vi "datearray_folder_creation.vi"(8 "error in":errorcluster, 11 "Cluster":T1={"path_Orig"=path "", "bo_Empty_Orig"=TRUE, "bo_exist_Orig"=TRUE, "path_Destin"=path "", "bo_Empty_Dest"=TRUE, "bo_exist_Dest"=TRUE, "bool_Erase"=FALSE, "arr_cl_lastmod_path"=[]}) -> (0 "error out":errorcluster, 3 "arr_copiedfiles":path[](array[path]))   [LabVIEW 2026]
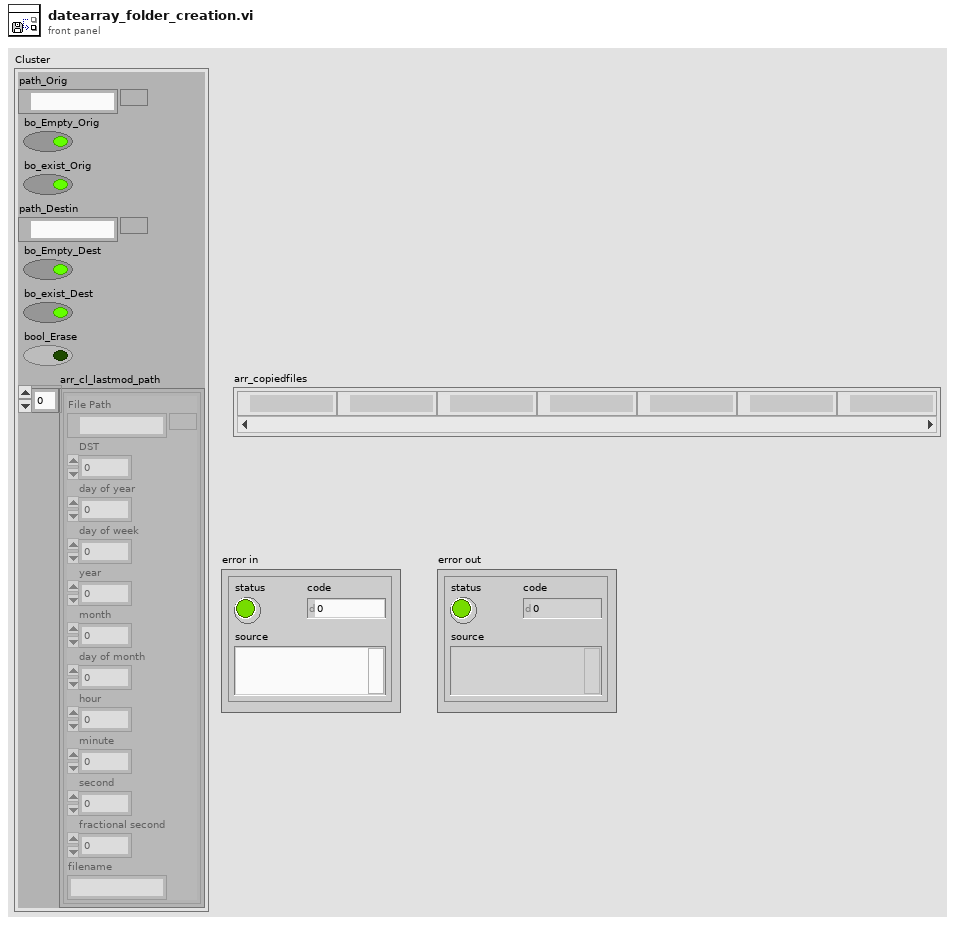
[diagram p1: front panel]
types:
  T1 = cluster{"path_Orig":path, "bo_Empty_Orig":bool, "bo_exist_Orig":bool, "path_Destin":path, "bo_Empty_Dest":bool, "bo_exist_Dest":bool, "bool_Erase":bool, "arr_cl_lastmod_path":cluster{"File Path":path, "DST":i32, "day of year":i32, "day of week":i32, "year":i32, "month":i32, "day of month":i32, "hour":i32, "minute":i32, "second":i32, "fractional second":dbl, "filename":string}[]}
  T2 = cluster{"File Path":path, "DST":i32, "day of year":i32, "day of week":i32, "year":i32, "month":i32, "day of month":i32, "hour":i32, "minute":i32, "second":i32, "fractional second":dbl, "filename":string}[]
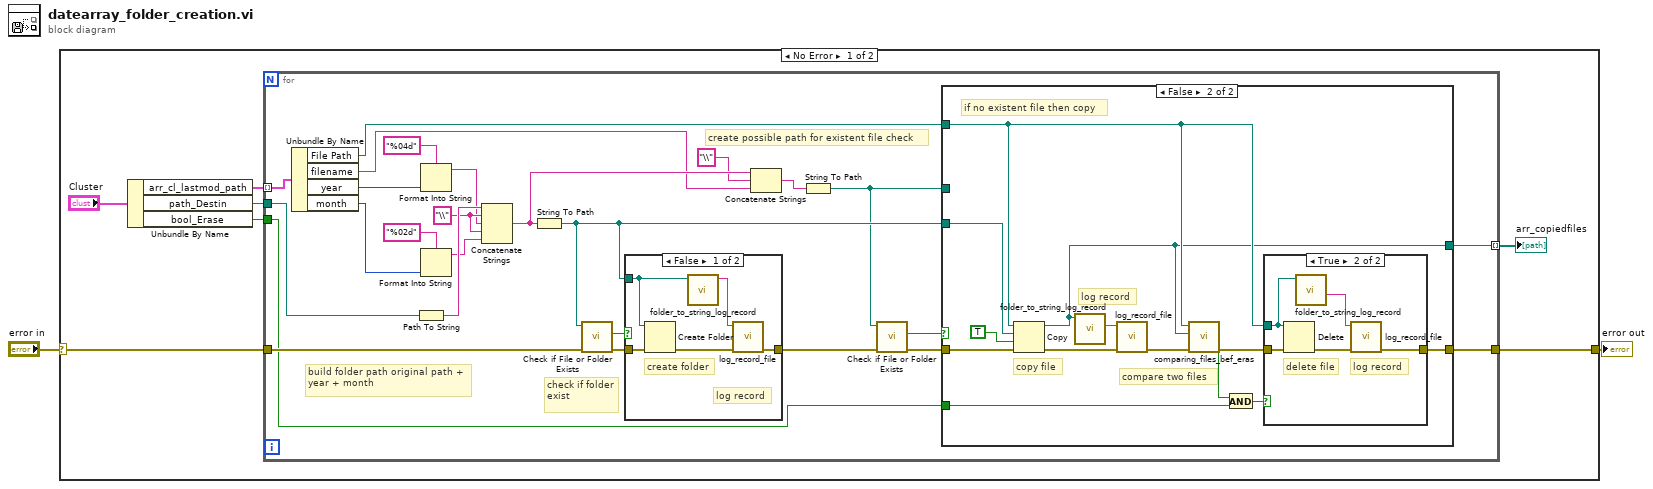
[diagram p0: block diagram]
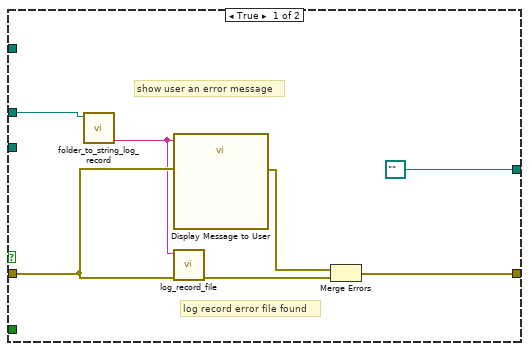
[diagram p2: hidden frame]
diagram:
  n1 = case shown="No Error" "error in" {
    selector: "error in" -> [w9 w68]
    tunnel: [w7 w68] -> w1
    frame No Error {
      n2 = Unbundle By Name("Cluster") -> ("arr_cl_lastmod_path"=w5:T2, "path_Destin"=w8:path, "bool_Erase"=w3:bool)
      n3 = for {
        tunnel: w8 -> [w34]
        tunnel: w9 -> [w32]
        tunnel: [w22] -> w7
        tunnel: [w20] -> w6 mode=indexing
        tunnel: w5 -> [w21] mode=indexing
        tunnel: w3 -> [w16]
        w33 = "\\"
        # "create possible path for existent file check"
        # "check if folder exist"
        # "build folder path original path + year + month"
        n4 = Unbundle By Name(w21) -> ("File Path"=w15:path, "filename"=w11:string, "year"=w26:i32, "month"=w29:i32)
        n5 = Path To String(path=w34) -> (string=w35:string)
        n6 = Format Into String(format string="%04d", w26) -> (resulting string=w25:string)  [unwired: 2 in, 1 out]
        n7 = Format Into String(format string="%02d", w29) -> (resulting string=w24:string)  [unwired: 2 in, 1 out]
        n8 = Concatenate Strings(w35, w33, w25, w33, w24) -> (w13:string)
        n9 = String To Path(string=w13) -> (path=w23:path)
        n10 = call <vilib>:"Check if File or Folder Exists.vi"("error in (no error)"=w32, "path"=w23) -> ("error out"=w30:errorcluster, "file or folder exists?"=w31:bool)  [unwired: 7 in, 1 out]
        n11 = case shown="False" w31 {
          tunnel: w30 -> [w66 w67]
          tunnel: [w64 w67] -> w19
          tunnel: w23 -> [w62 _]
          frame False {
            # "log record"
            # "create folder"
            n12 = Create Folder(path (use dialog)=w62, error in=w66) -> (error out=w65:errorcluster)  [unwired: 1 in, 2 out]
            n13 = call "folder_to_string_log_record.vi"("File Path"=w62) -> ("str_foldercreat"=w63:string)  [unwired: 7 in, 3 out]
            n14 = call "log_record_file.vi"("error in"=w65, "st_LogEvent"=w63) -> ("error out"=w64:errorcluster)  [unwired: 9 in]
          }
          frame True {
          }
        }
        n15 = Concatenate Strings(w13, "\\", w11) -> (w14:string)
        n16 = String To Path(string=w14) -> (path=w10:path)
        n17 = call <vilib>:"Check if File or Folder Exists.vi"("error in (no error)"=w19, "path"=w10) -> ("error out"=w18:errorcluster, "file or folder exists?"=w17:bool)  [unwired: 7 in, 1 out]
        n18 = case shown="False" w17 {
          tunnel: w18 -> [w40 w55]
          tunnel: w23 -> [_ w53]
          tunnel: [w41 w52] -> w22
          tunnel: w15 -> [_ w47]
          tunnel: [path "" ("new path") w46] -> w20
          tunnel: w16 -> [_ w49]
          tunnel: w10 -> [w38 _]
          frame True {
            # "show user an error message"
            # "log record error file found"
            n19 = call "folder_to_string_log_record.vi"("File Path"=w38) -> ("str_fileerrror"=w37:string)  [unwired: 7 in, 3 out]
            n20 = call "Display Message to User"("error in (no error)"=w40, "Message"=w37) -> ("error out"=w39:errorcluster)  [unwired: 8 in, 1 out]
            n21 = call "log_record_file.vi"("error in"=w40, "st_LogEvent"=w37) -> ("error out"=w42:errorcluster)  [unwired: 9 in]
            n22 = Merge Errors(w39, w42) -> (w41:errorcluster)
          }
          frame False {
            # "compare two files"
            # "if no existent file then copy"
            # "log record"
            # "copy file"
            n23 = Copy(8:w55, 9:TRUE, 10:w53, 11:w47) -> (0:w51:errorcluster, 3:w46:path)  [unwired: 1 in, 1 out]
            n24 = call "folder_to_string_log_record.vi"("File Path"=w46) -> ("str_filecopyed"=w50:string)  [unwired: 7 in, 3 out]
            n25 = call "log_record_file.vi"("error in"=w51, "st_LogEvent"=w50) -> ("error out"=w44:errorcluster)  [unwired: 9 in]
            n26 = call "comparing_files_bef_eras.vi"("error in"=w44, "path_filecopied"=w46, "path_fileorigin"=w47) -> ("error out"=w43:errorcluster, "bol_equals"=w45:bool)  [unwired: 7 in]
            n27 = And(x=w45, y=w49) -> (x .and. y?=w48:bool)
            n28 = case shown="True" w48 {
              tunnel: [w56 w59] -> w52
              tunnel: w43 -> [w56 w61]
              tunnel: w47 -> [_ w57]
              frame False {
              }
              frame True {
                # "log record"
                # "delete file"
                n29 = Delete(path (use dialog)=w57, error in=w61) -> (error out=w60:errorcluster)  [unwired: 3 in, 2 out]
                n30 = call "folder_to_string_log_record.vi"("File Path"=w57) -> ("str_fileerased"=w58:string)  [unwired: 7 in, 3 out]
                n31 = call "log_record_file.vi"("error in"=w60, "st_LogEvent"=w58) -> ("error out"=w59:errorcluster)  [unwired: 9 in]
              }
            }
          }
        }
      }
      "arr_copiedfiles" <- w6
    }
    frame Error {
    }
  }
  "error out" <- w1
